vi "Kinect Depth Controler.vi"(9 "y":dbl, 10 "x":dbl) -> ()   [LabVIEW 2015]
uses:
  subVIs/Video Resolution Control.ctl
  subVIs/Video Format Control.ctl
  subVIs/Depth Format Control.ctl
  subVIs/Depth Resolution Control.ctl
  subVIs/Led Control.ctl
  subVIs/Log Level Control.ctl
panel:
  in  "stop":bool
  out "y":dbl
  out "x":dbl
  out "error out":errorcluster
  in  "Led Option":T1=enum."LED_RED"
  in  "Video & Depth Config":T6
  in  "Tilt degree":i32=5 min=-28 max=28
  out "Depth image":picture
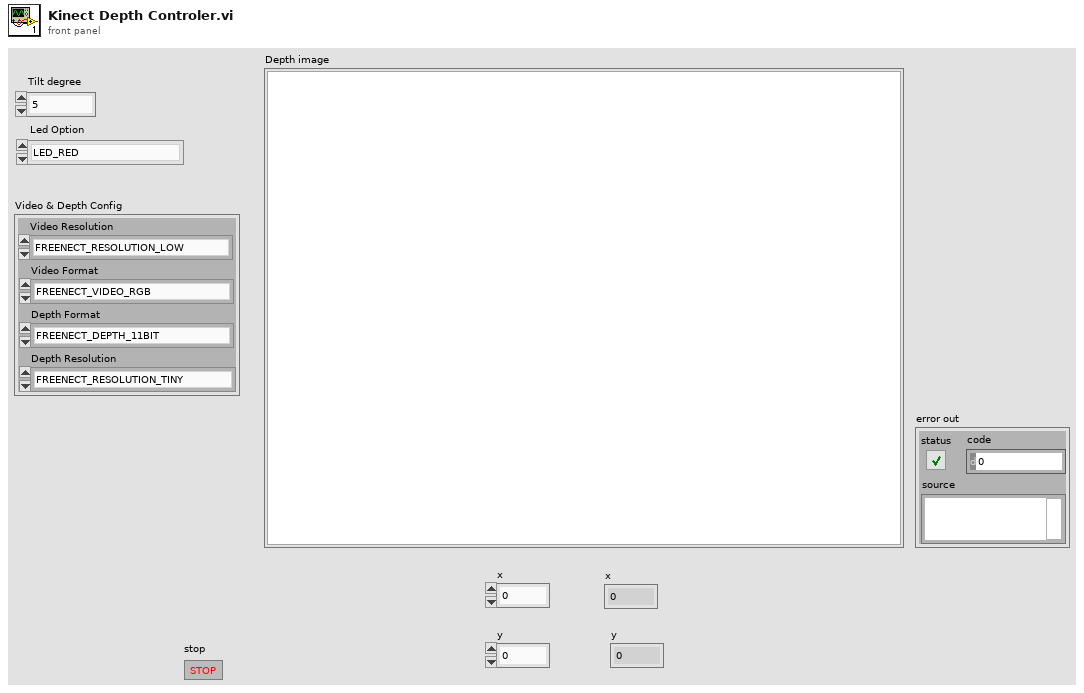
[diagram p1: front panel]
types:
  T1 = typedef "Led Control.ctl" = enum32{"LED_OFF", "LED_GREEN", "LED_RED", "LED_YELLOW", "LED_BLINK_GREEN", "LED_BLINK_GREEN2", "LED_BLINK_RED_YELLOW"}
  T2 = typedef "Video Resolution Control.ctl" = enum32{"FREENECT_RESOLUTION_LOW", "FREENECT_RESOLUTION_MEDIUM", "FREENECT_RESOLUTION_HIGH"}
  T3 = typedef "Video Format Control.ctl" = enum32{"FREENECT_VIDEO_RGB", "FREENECT_VIDEO_BAYER", "FREENECT_VIDEO_IR_8BIT", "FREENECT_VIDEO_IR_10BIT", "FREENECT_VIDEO_IR_10BIT_PACKED", "FREENECT_VIDEO_YUV_RGB", "FREENECT_VIDEO_YUV_RAW"}
  T4 = typedef "Depth Format Control.ctl" = enum32{"FREENECT_DEPTH_11BIT", "FREENECT_DEPTH_10BIT", "FREENECT_DEPTH_11BIT_PACKED", "FREENECT_DEPTH_10BIT_PACKED", "FREENECT_DEPTH_REGISTERED", "FREENECT_DEPTH_MM"}
  T5 = typedef "Depth Resolution Control.ctl" = enum16{"FREENECT_RESOLUTION_TINY", "FREENECT_RESOLUTION_LOW", "FREENECT_RESOLUTION_MEDIUM"}
  T6 = cluster{"Video Resolution":T2, "Video Format":T3, "Depth Format":T4, "Depth Resolution":T5}
  T7 = typedef "Log Level Control.ctl" = enum32{"FREENECT_LOG_FATAL", "FREENECT_LOG_ERROR", "FREENECT_LOG_WARNING", "FREENECT_LOG_NOTICE", "FREENECT_LOG_INFO", "FREENECT_LOG_DEBUG", "FREENECT_LOG_SPEW", "FREENECT_LOG_FLOOD"}
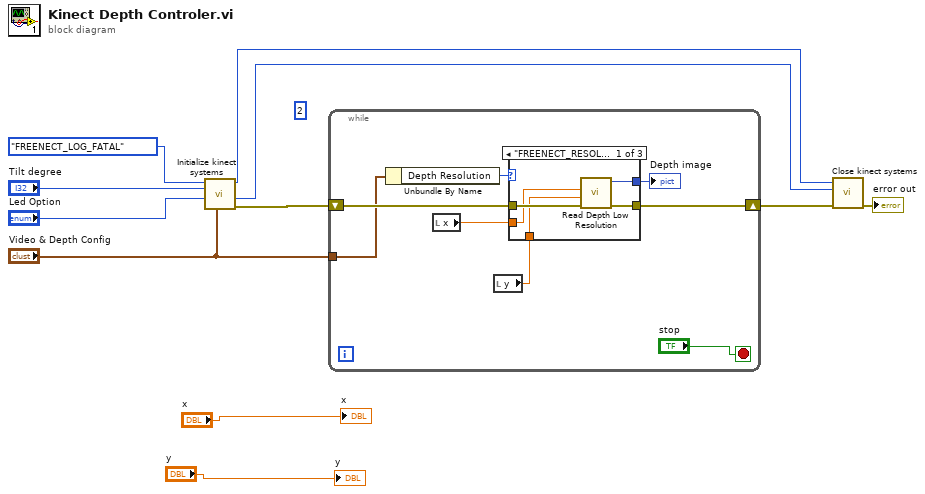
[diagram p0: block diagram]
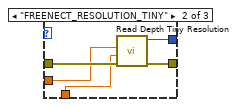
[diagram p2: hidden frame]
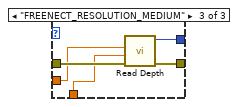
[diagram p3: hidden frame]
diagram:
  (unwired) 2
  n1 = call "Initialize kinect systems.vi"("Video and Depth config"="Video & Depth Config", "Led Option"="Led Option", "tilt degree"="Tilt degree", "Log Level"=Log_Level_Control."FREENECT_LOG_FATAL") -> ("error out"=w10:errorcluster, "Kinect Handle"=w9:i64, "Video Handle out"=w3:i64)  [unwired: 4 in, 1 out]
  n2 = while {
    tunnel: "Video & Depth Config" -> [w17]
    shift-right: [w19] -> w11
    shift-left: w10 -> [w18]
    stop <- "stop" stop-if-true
    n3 = Unbundle By Name(w17) -> ("Depth Resolution"=w15:T5)
    n4 = local read "x"() -> (w14:dbl)
    n5 = local read "y"() -> (w13:dbl)
    n6 = case shown="\"FREENECT_RESOLUTION_LOW\", Default" w15 {
      tunnel: w18 -> [w24 w27 w34]
      tunnel: [w23 w28 w33] -> w19
      tunnel: [w22 w29 w32] -> w16
      tunnel: w14 -> [w21 w26 w31]
      tunnel: w13 -> [w20 w25 w30]
      frame "FREENECT_RESOLUTION_LOW", Default {
        n7 = call "Read Depth Low Resolution.vi"("error in (no error)"=w24, "y"=w20, "x"=w21) -> ("error out"=w23:errorcluster, "Depth image"=w22:picture)  [unwired: 7 in]
      }
      frame "FREENECT_RESOLUTION_TINY" {
        n8 = call "Read Depth Tiny Resolution.vi"("error in (no error)"=w27, "y"=w25, "x"=w26) -> ("error out"=w28:errorcluster, "Depth image"=w29:picture)  [unwired: 7 in]
      }
      frame "FREENECT_RESOLUTION_MEDIUM" {
        n9 = call "Read Depth.vi"("error in (no error)"=w34, "y"=w30, "x"=w31) -> ("error out"=w33:errorcluster, "Depth image"=w32:picture)  [unwired: 7 in]
      }
    }
    "Depth image" <- w16
  }
  n10 = call "Close kinect systems.vi"("error in (no error)"=w11, "Kinect Handle"=w9, "Video handle in"=w3) -> ("error out"=→"error out":errorcluster)  [unwired: 8 in]
  "x" <- "x"
  "y" <- "y"
